vi "In Range and Coerce.vi"() -> ()   [LabVIEW 2023]
doc: "This example shows how the In Range and Coerce function operates with different data types."
panel:
  in  "Tab Control":T1(tab)
  in  "Lower Limit":dbl=5.0
  in  "Upper Limit":dbl=87.0
  out "Coerced Numeric":dbl
  out "Numeric in Range?":bool
  in  "Numeric":dbl=47.0
  out "Coerced String":string
  out "String in Range?":bool
  in  "String":string="B"
  in  "Lower Limit":string="A"
  in  "Upper Limit":string="C"
  out "Cluster in Range?":T2
  out "Coerced Cluster":T3
  in  "Lower Limit":dbl=4.0
  in  "Upper Limit":dbl=6.0
  in  "Cluster":T3={"Numeric 1"=7.0, "Numeric 2"=5.0, "Numeric 3"=3.0}
  out "Aggregate Cluster in Range?":bool
  in  "Lower Limits":T3={"Numeric 1"=75.0, "Numeric 2"=52.0, "Numeric 3"=81.0}
  in  "Upper Limits":T3={"Numeric 1"=100.0, "Numeric 2"=57.0, "Numeric 3"=99.0}
  in  "Cluster":T3={"Numeric 1"=78.0, "Numeric 2"=59.0, "Numeric 3"=87.0}
  out "Array in Range?":bool[](array[boolean])
  out "Coerced Array":dbl[](array[numeric])
  in  "Lower Limit":dbl=2.0
  in  "Upper Limit":dbl=5.0
  in  "Input Array":dbl[](array[numeric])=[1.0, 2.0, 3.0, 4.0, 5.0]
  out "Aggregate Array in Range?":bool
  in  "Upper Limit":dbl[](array[numeric])=[3.0, 3.0, 4.0, 4.0, 5.0]
  in  "Lower Limit":dbl[](array[numeric])=[0.0, 0.0, 1.0, 1.0, 2.0]
  in  "Input Array":dbl[](array[numeric])=[1.0, 2.0, 3.0, 4.0, 5.0]
  # "Overview: Demonstrates how the In Range and Coerce function operates with different data types.\nInstructions:\n1. Run the VI.\n2. Examine the different cases."
  # "Check the Numeric value against the specified upper and lower limits."
  # "In Range and Coerce checks strings based on their ASCII numeric values, which means that the range check on strings is case sensitive."
  # "With clusters in Compare Elements mode, each value in the cluster is checked against the specified limits, with a cluster of Booleans returned for the In Range? result."
  # "With clusters in Compare Aggregates mode, only the first element in the cluster is checked against the range defined by the first elements in the upper and lower limit clusters."
  # "With arrays in Compare Elements mode, each value in the array is checked against the specified limits, with an array of Booleans returned for the In Range? result."
  # "With arrays in Compare Aggregates mode, only the first element in the array is checked against the range defined by the first elements in the upper and lower limit arrays."
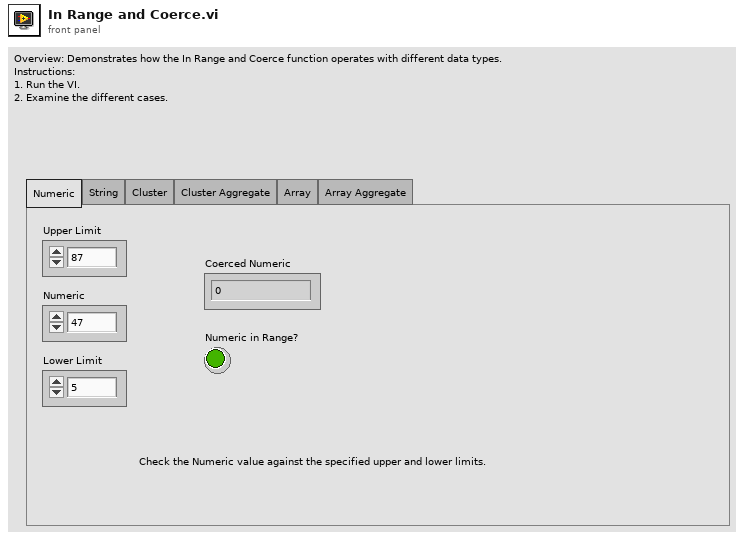
[diagram p1: front panel]
types:
  T1 = enum32{"Numeric", "String", "Cluster", "Cluster Aggregate", "Array", "Array Aggregate"}
  T2 = cluster{"Numeric 1":bool, "Numeric 2":bool, "Numeric 3":bool}
  T3 = cluster{"Numeric 1":dbl, "Numeric 2":dbl, "Numeric 3":dbl}
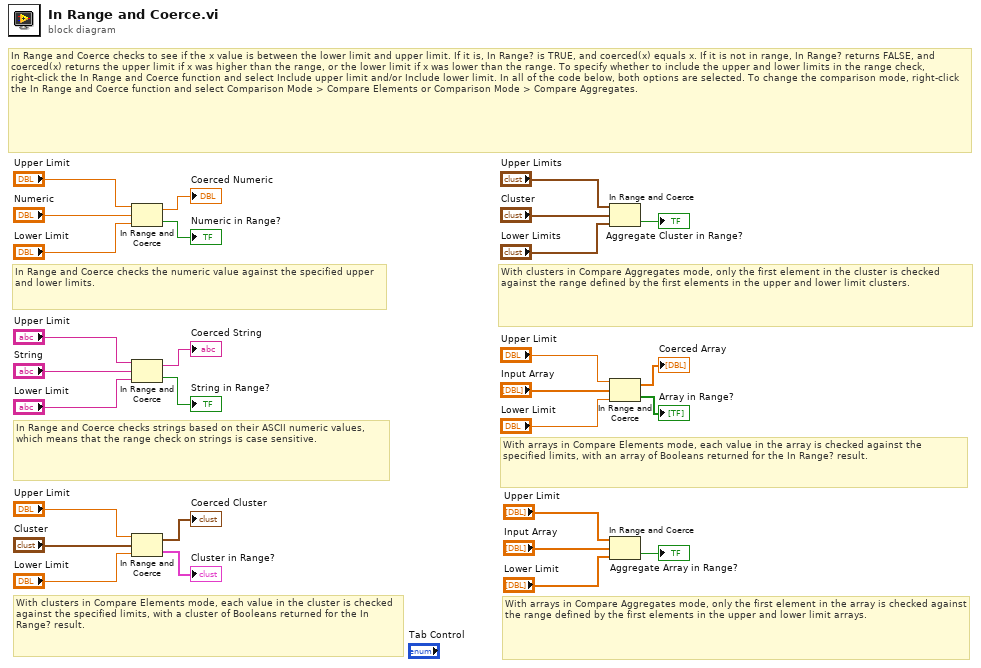
[diagram p0: block diagram]
diagram:
  # "With arrays in Compare Elements mode, each value in the array is checked against the specified limits, with an array of Booleans returned for the In Range? result."
  # "In Range and Coerce checks to see if the x value is between the lower limit and upper limit. If it is, In Range? is TRUE, and coerced(x) equals x. If it is not in range, In Range? returns FALSE, and coerced(x) returns the upper limit if x was higher than the range, or the lower limit if x was lower than the range. To specify whether to include the upper and lower limits in the range check, right-click the In Range and Coerce function and select Include upper limit and/or Include lower limit. In all of the code below, both options are selected. To change the comparison mode, right-click the In Range and Coerce function and select Comparison Mode > Compare Elements or Comparison Mode > Compare Aggregates."
  # "In Range and Coerce checks strings based on their ASCII numeric values, which means that the range check on strings is case sensitive."
  # "With clusters in Compare Elements mode, each value in the cluster is checked against the specified limits, with a cluster of Booleans returned for the In Range? result."
  # "With clusters in Compare Aggregates mode, only the first element in the cluster is checked against the range defined by the first elements in the upper and lower limit clusters."
  # "With arrays in Compare Aggregates mode, only the first element in the array is checked against the range defined by the first elements in the upper and lower limit arrays."
  # "In Range and Coerce checks the numeric value against the specified upper and lower limits."
  n1 = In Range and Coerce(upper limit="Upper Limit", x="Numeric", lower limit="Lower Limit") -> (coerced(x)=→"Coerced Numeric":dbl, In Range?=→"Numeric in Range?":bool)
  n2 = In Range and Coerce(upper limit="Upper Limit", x="String", lower limit="Lower Limit") -> (coerced(x)=→"Coerced String":string, In Range?=→"String in Range?":bool)
  n3 = In Range and Coerce(upper limit="Upper Limit", x="Cluster", lower limit="Lower Limit") -> (coerced(x)=→"Coerced Cluster":T3, In Range?=→"Cluster in Range?":T2)
  n4 = In Range and Coerce(upper limit="Upper Limits", x="Cluster", lower limit="Lower Limits") -> (In Range?=→"Aggregate Cluster in Range?":bool)  [unwired: 1 out]
  n5 = In Range and Coerce(upper limit="Upper Limit", x="Input Array", lower limit="Lower Limit") -> (coerced(x)=→"Coerced Array":dbl[], In Range?=→"Array in Range?":bool[])
  n6 = In Range and Coerce(upper limit="Upper Limit", x="Input Array", lower limit="Lower Limit") -> (In Range?=→"Aggregate Array in Range?":bool)  [unwired: 1 out]
